vi "ULx Create Channel (CO-Pulse Generation-Frequency).vi"(0 "task in":refnum<k24>, 1 "frequency":dbl=1.0 format="%.6f", 2 "duty cycle":dbl=0.5 format="%.6f", 5 "counters":refnum<k21>, 11 "error in":errorcluster) -> (4 "task out":refnum<k24>, 15 "error out":errorcluster)   [LabVIEW 2020]
doc: "Creates channel(s) to generate digital pulses that frequency and duty cycle define."
uses:
  C:/Users/William/Documents/LV 2020 builds/LeaktestDAQ/Source-v33/ULx_LV.dll
  ULx_LV.dll
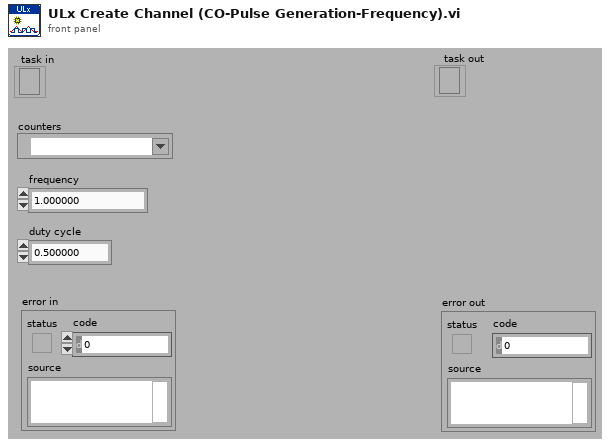
[diagram p1: front panel]
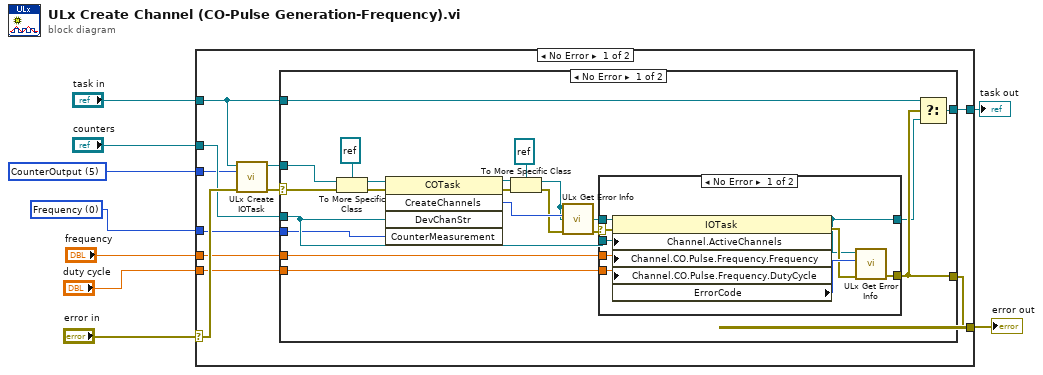
[diagram p0: block diagram]
diagram:
  w3 = 0 items=["Frequency", "Time", "Ticks"] ("RateGenerationType")
  w5 = 5 items=["AnalogInput", "AnalogOutput", "DigitalInput", "DigitalOutput", "CounterInput", "CounterOutput", "CompositeInput", "CompositeOutput", "TemperatureInput"] ("taskType")
  n1 = case shown="No Error" "error in" {
    selector: "error in" -> [w20 w55]
    tunnel: "task in" -> [w10 w54]
    tunnel: "counters" -> [w15 _]
    tunnel: [w18 w54] -> w7
    tunnel: [w17 w55] -> w6
    tunnel: w5 -> [w14 _]
    tunnel: w3 -> [w13 _]
    tunnel: "frequency" -> [w12 _]
    tunnel: "duty cycle" -> [w11 _]
    frame No Error {
      n2 = call "ULx Create IOTask.vi"("error in"=w20, "taskType"=w14, "i/o task in"=w10) -> ("error out"=w19:errorcluster, "i/o task out"=w16:refnum<k24>)  [unwired: 7 in]
      n3 = case shown="No Error" w19 {
        selector: w19 -> [w38 w53]
        tunnel: [w22 w53] -> w17
        tunnel: [w24 w52] -> w18
        tunnel: w16 -> [w36 _]
        tunnel: w15 -> [w33 _]
        tunnel: w13 -> [w32 _]
        tunnel: w12 -> [w31 _]
        tunnel: w11 -> [w30 _]
        tunnel: w10 -> [w23 w52]
        frame No Error {
          n4 = To More Specific Class(target class=refnum<k24> refnum, reference=w36, error in=w38) -> (specific class reference=w39:refnum<k24>, error out=w37:errorcluster)
          n5 = invoke class="COTask" method="CreateChannels"(reference=w39, error in=w37, "DevChanStr"=w33, "CounterMeasurement"=w32) -> (reference out=w28:refnum<k24>, error out=w27:errorcluster, "CreateChannels"=w35:i32)  [unwired: 1 in, 2 out]
          n6 = To More Specific Class(target class=refnum<k24> refnum, reference=w28, error in=w27) -> (specific class reference=w25:refnum<k24>, error out=w26:errorcluster)
          n7 = call "ULx Get Error Info.vi"("error in"=w26, "ErrorCode"=w35, "task in"=w25) -> ("error out"=w34:errorcluster)  [unwired: 8 in]
          n8 = case shown="No Error" w34 {
            selector: w34 -> [w49 w51]
            tunnel: w25 -> [w48 w50]
            tunnel: w33 -> [w47 _]
            tunnel: [w44 w51] -> w22
            tunnel: w31 -> [w43 _]
            tunnel: w30 -> [w42 _]
            tunnel: [w41 w50] -> w21
            frame No Error {
              n9 = property class="IOTask"(reference=w48, error in=w49, "Channel.ActiveChannels"=w47, "Channel.CO.Pulse.Frequency.Frequency"=w43, "Channel.CO.Pulse.Frequency.DutyCycle"=w42) -> (reference out=w41:refnum<k24>, error out=w45:errorcluster, "ErrorCode"=w46:i32)
              n10 = call "ULx Get Error Info.vi"("error in"=w45, "ErrorCode"=w46, "task in"=w41) -> ("error out"=w44:errorcluster)  [unwired: 8 in]
            }
            frame Error {
            }
          }
          n11 = Select(t=w23, s=w22, f=w21) -> (s? t:f=w24:refnum<k24>)
        }
        frame Error {
        }
      }
    }
    frame Error {
    }
  }
  "error out" <- w6
  "task out" <- w7
